vi "Log (Log Record).vi"(10 "log record":T1 {"timestamp" format="%<%x %.3X>T"}, 11 "Logger in":refnum<class "Logger.lvclass">) -> (3 "Logger out":refnum<class "Logger.lvclass">)   [LabVIEW 2018, in "GLog.lvlib" / "Logger.lvclass"]
uses:
  Logger.lvclass
  Log Record.ctl
  Internal Log Levels.ctl
  Logger.lvclass/Logger.ctl
  extension/scope_interface/Scope.lvclass
  extension/filter_interface/Filter.lvclass
  GLog.lvlib
panel:
  # "Connector Pane"
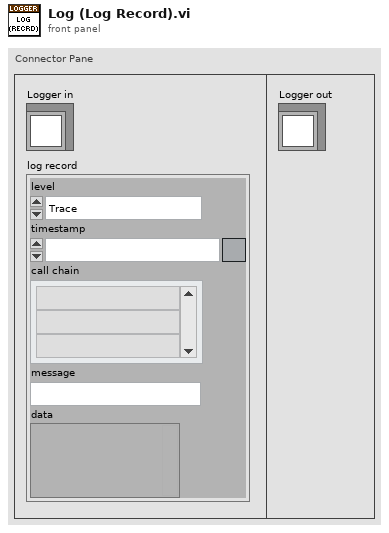
[diagram p1: front panel]
types:
  T1 = typedef "GLog.lvlib/Log Record.ctl" = cluster{"level":T2, "timestamp":timestamp, "call chain":string[], "message":string, "data":variant}
  T2 = typedef "GLog.lvlib/Internal Log Levels.ctl" = enum16{"Trace", "Debug", "Info", "Warning", "Error", "Critical", "Internal"}
  T3 = typedef "GLog.lvlib/Log Levels.ctl" = enum16{"Trace", "Debug", "Info", "Warning", "Error", "Critical"}
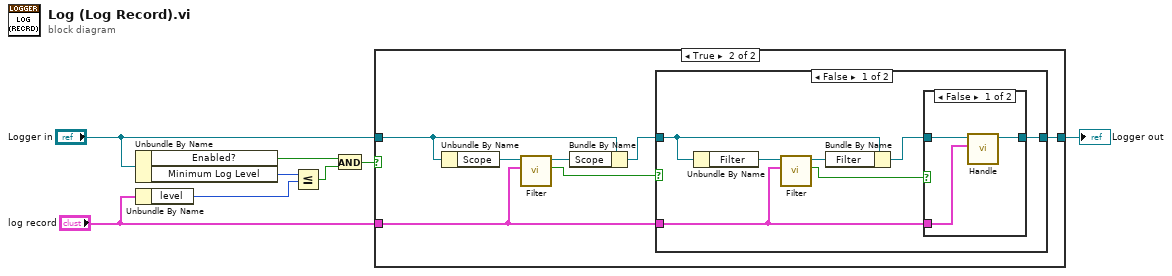
[diagram p0: block diagram]
diagram:
  n1 = Unbundle By Name("Logger in") -> ("Enabled?"=w2:bool, "Minimum Log Level"=w3:T3)
  n2 = Unbundle By Name("log record") -> ("level"=w8:T2)
  n3 = Less Or Equal?(x=w3, y=w8) -> (x <= y?=w4:bool)
  n4 = And(x=w2, y=w4) -> (x .and. y?=w1:bool)
  n5 = case shown="True" w1 {
    tunnel: [w9 w13] -> w6
    tunnel: "log record" -> [_ w10]
    tunnel: "Logger in" -> [w9 w12]
    frame False {
    }
    frame True {
      n6 = Unbundle By Name(w12) -> ("Scope"=w16:refnum<class "Scope.lvclass">)
      n7 = call-dynamic "Filter.vi"("log record"=w10, "filter in"=w16) -> ("discard?"=w11:bool, "filter out"=w15:refnum<class "Scope.lvclass">)  [unwired: 8 in]
      n8 = Bundle By Name(cluster=w12, "Scope"=w15) -> (w14:refnum<class "Logger.lvclass">)
      n9 = case shown="False" w11 {
        tunnel: w14 -> [w23 w28]
        tunnel: [w19 w28] -> w13
        tunnel: w10 -> [w18 _]
        frame False {
          n10 = Unbundle By Name(w23) -> ("Filter"=w22:refnum<class "Filter.lvclass">)
          n11 = call-dynamic "Filter.vi"("log record"=w18, "filter in"=w22) -> ("discard?"=w17:bool, "filter out"=w21:refnum<class "Filter.lvclass">)  [unwired: 8 in]
          n12 = Bundle By Name(cluster=w23, "Filter"=w21) -> (w20:refnum<class "Logger.lvclass">)
          n13 = case shown="False" w17 {
            tunnel: w20 -> [w24 w27]
            tunnel: [w26 w27] -> w19
            tunnel: w18 -> [w25 _]
            frame False {
              n14 = call "Handle.vi"("log record"=w25, "logger in"=w24) -> ("logger out"=w26:refnum<class "Logger.lvclass">)  [unwired: 9 in]
            }
            frame True {
            }
          }
        }
        frame True {
        }
      }
    }
  }
  "Logger out" <- w6
